vi "P&T_Plot Labels.vi"(7 "Plots FGV Control":enum16{"Get Text", "Pass Text", "Write Text"}(ring), 8 "Error In":errorcluster) -> (0 "Error Out":errorcluster, 3 "Array":string[](array[string]))   [LabVIEW 2016]
uses:
  DAQLoop_Typedef.ctl
panel:
  in  "Cluster":T1
  out "appended path":path
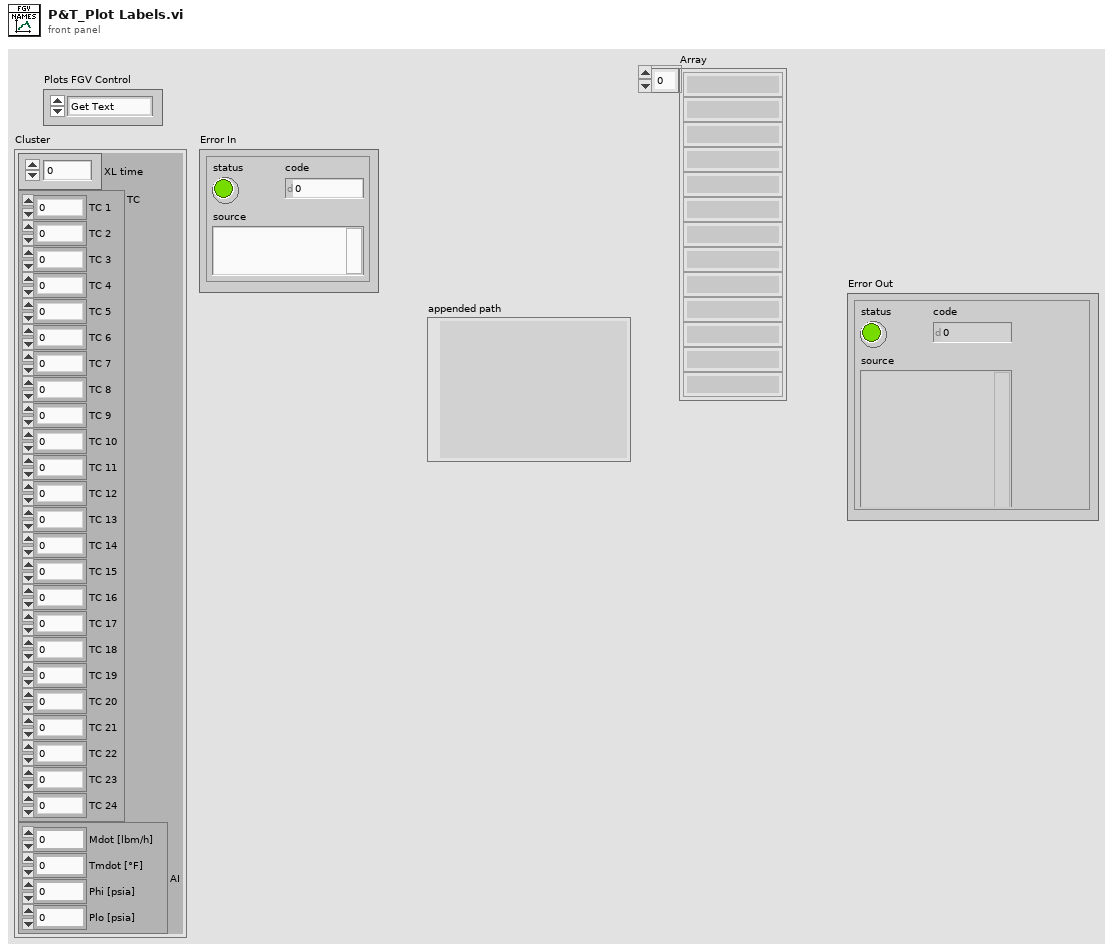
[diagram p1: front panel]
types:
  T1 = typedef "DAQLoop_Typedef.ctl" = cluster{"XL time":dbl, "TC":cluster{"TC 1":dbl, "TC 2":dbl, "TC 3":dbl, "TC 4":dbl, "TC 5":dbl, "TC 6":dbl, "TC 7":dbl, "TC 8":dbl, "TC 9":dbl, "TC 10":dbl, "TC 11":dbl, "TC 12":dbl, "TC 13":dbl, "TC 14":dbl, "TC 15":dbl, "TC 16":dbl, "TC 17":dbl, "TC 18":dbl, "TC 19":dbl, "TC 20":dbl, "TC 21":dbl, "TC 22":dbl, "TC 23":dbl, "TC 24":dbl}, "AI":cluster{"Mdot [lbm/h]":dbl, "Tmdot [°F]":dbl, "Phi [psia]":dbl, "Plo [psia]":dbl}}
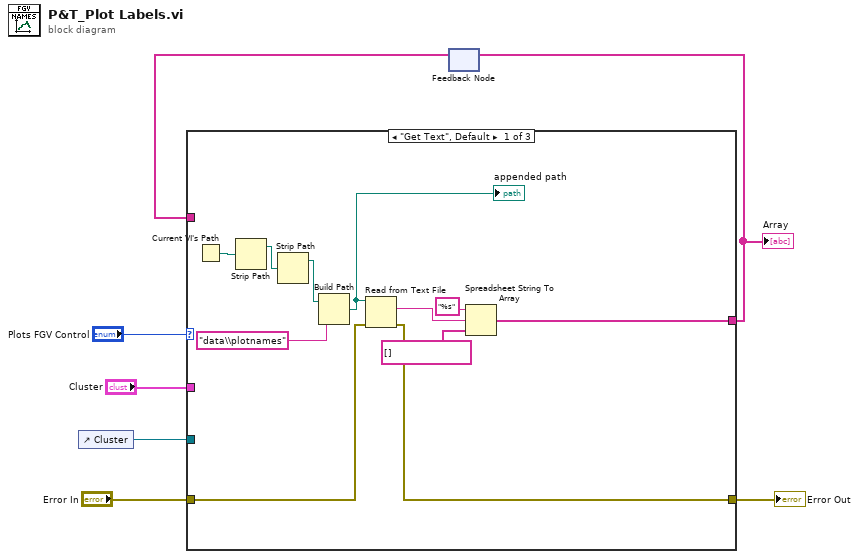
[diagram p0: block diagram]
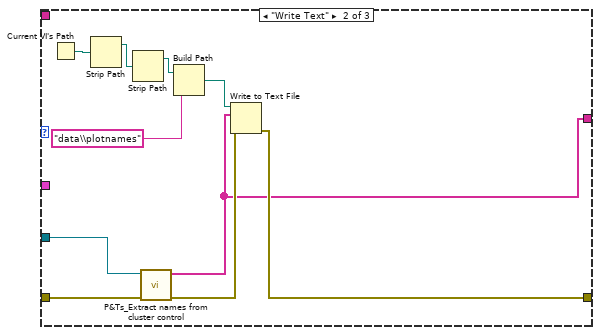
[diagram p2: hidden frame]
diagram:
  n1 = control-ref of="Cluster"() -> (w3:refnum<vi>)
  n2 = feedback #1() -> (w5:string[])  [unwired: 1 in]
  n3 = case shown="\"Get Text\", Default" "Plots FGV Control" {
    tunnel: [w14 w19 w30] -> w6
    tunnel: w5 -> [_ _ w30]
    tunnel: "Cluster" -> [_ _ _]
    tunnel: w3 -> [_ w23 _]
    tunnel: "Error In" -> [w10 w22 w29]
    tunnel: [w9 w20 w29] -> w1
    frame "Get Text", Default {
      n4 = Current VI's Path() -> (path=w18:path)
      n5 = Strip Path(path=w18) -> (stripped path=w13:path)  [unwired: 1 out]
      n6 = Strip Path(path=w13) -> (stripped path=w12:path)  [unwired: 1 out]
      n7 = Build Path(base path=w12, name or relative path="data\\plotnames") -> (appended path=w11:path)
      "appended path" <- w11
      n8 = Read from Text File(file (use dialog)=w11, error in=w10) -> (text=w8:string, error out=w9:errorcluster)  [unwired: 2 in, 2 out]
      n9 = Spreadsheet String To Array(format string="%s", spreadsheet string=w8, array type (2D Dbl)=string[] [] ("Array")) -> (array=w14:string[])  [unwired: 1 in]
    }
    frame "Write Text" {
      n10 = Current VI's Path() -> (path=w28:path)
      n11 = Strip Path(path=w28) -> (stripped path=w26:path)  [unwired: 1 out]
      n12 = Strip Path(path=w26) -> (stripped path=w25:path)  [unwired: 1 out]
      n13 = call "P&Ts_Extract names from cluster control.vi"("error in (no error)"=w22, "Cluster In"=w23) -> ("error out"=w21:errorcluster, "Array"=w19:string[])  [unwired: 8 in]
      n14 = Build Path(base path=w25, name or relative path="data\\plotnames") -> (appended path=w24:path)
      n15 = Write to Text File(file (use dialog)=w24, text=w19, error in=w21) -> (error out=w20:errorcluster)  [unwired: 1 in, 2 out]
    }
    frame "Pass Text" {
    }
  }
  "Array" <- w6
  "Error Out" <- w1
  n16 = feedback-in #1(w6) -> ()
